vi "Delta_theta.vi"(9 "delta_L":dbl, 10 "etta":dbl) -> (2 "Delta_theta":dbl)   [LabVIEW 2014]
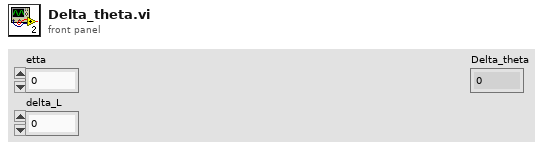
[diagram p1: front panel]
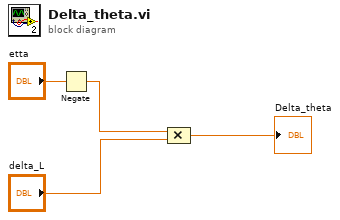
[diagram p0: block diagram]
diagram:
  n1 = Negate(x="etta") -> (-x=w2:dbl)
  n2 = Compound Arithmetic op=MULTIPLY(w2, "delta_L") -> (→"Delta_theta":dbl)
